vi "Operational Dashboard Send.vi"(10 "Robot Commands":T1) -> ()   [LabVIEW 2014]
uses:
  Robot Commands.ctl
  <vilib>/Rock Robotics/Network Tables/SD Write Boolean Array.vi
  <vilib>/Rock Robotics/Network Tables/SD Write Boolean.vi
panel:
  # "Field Centric"
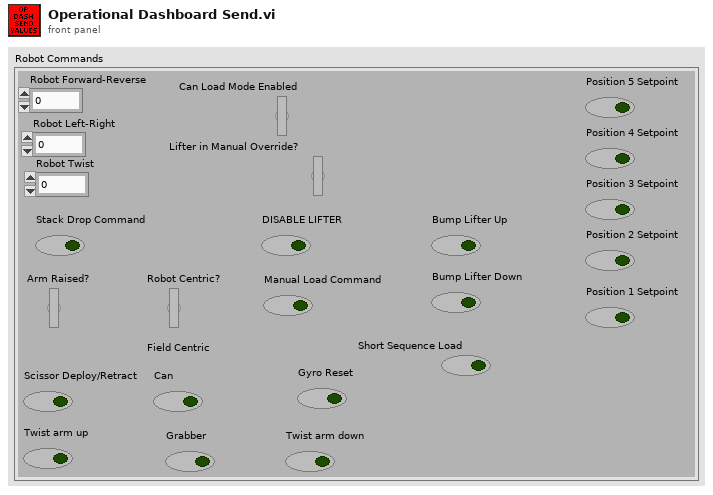
[diagram p1: front panel]
types:
  T1 = typedef "Robot Commands.ctl" = cluster{"Robot Forward-Reverse":dbl, "Robot Left-Right":dbl, "Robot Twist":dbl, "Can Load Mode Enabled":bool, "Lifter in Manual Override?":bool, "Stack Drop Command":bool, "Arm Raised?":bool, "DISABLE LIFTER":bool, "Position 1 Setpoint":bool, "Position 2 Setpoint":bool, "Position 3 Setpoint":bool, "Position 4 Setpoint":bool, "Position 5 Setpoint":bool, "Bump Lifter Down":bool, "Bump Lifter Up":bool, "Manual Load Command":bool, "Robot Centric?":bool, "Scissor Deploy/Retract":bool, "Grabber":bool, "Can":bool, "Twist arm up":bool, "Gyro Reset":bool, "Twist arm down":bool, "Short Sequence Load":bool}
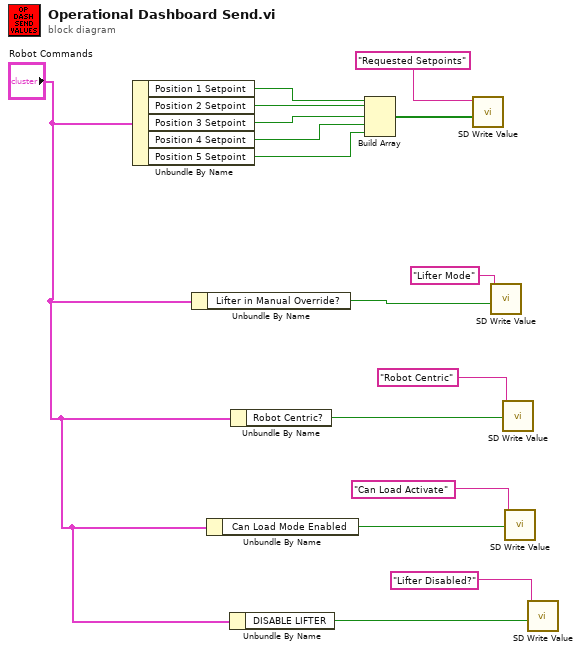
[diagram p0: block diagram]
diagram:
  n1 = Unbundle By Name("Robot Commands") -> ("Position 1 Setpoint"=w16:bool, "Position 2 Setpoint"=w15:bool, "Position 3 Setpoint"=w14:bool, "Position 4 Setpoint"=w13:bool, "Position 5 Setpoint"=w12:bool)
  n2 = Unbundle By Name("Robot Commands") -> ("Lifter in Manual Override?"=w9:bool)
  n3 = Unbundle By Name("Robot Commands") -> ("Can Load Mode Enabled"=w5:bool)
  n4 = Unbundle By Name("Robot Commands") -> ("DISABLE LIFTER"=w1:bool)
  n5 = Unbundle By Name("Robot Commands") -> ("Robot Centric?"=w7:bool)
  n6 = Build Array(w16, w15, w14, w13, w12) -> (w11:bool[])
  n7 = call-poly <vilib>:"SD Write Value.vi"("Boolean Array"=w11, "Name"="Requested Setpoints") -> ()  [unwired: 8 in, 2 out]
  n8 = call-poly <vilib>:"SD Write Value.vi"("Boolean"=w9, "Name"="Lifter Mode") -> ()  [unwired: 8 in, 2 out]
  n9 = call-poly <vilib>:"SD Write Value.vi"("Boolean"=w7, "Name"="Robot Centric") -> ()  [unwired: 8 in, 2 out]
  n10 = call-poly <vilib>:"SD Write Value.vi"("Boolean"=w5, "Name"="Can Load Activate") -> ()  [unwired: 8 in, 2 out]
  n11 = call-poly <vilib>:"SD Write Value.vi"("Boolean"=w1, "Name"="Lifter Disabled?") -> ()  [unwired: 8 in, 2 out]
